vi "Initialize.vi"(8 "error in (no error)":errorcluster, 9 "Reset? ( Yes)":bool=TRUE, 10 "ID Query? ( Yes)":bool=TRUE, 11 "VISA resource name":refnum<visa-resource-name>) -> (0 "error out":errorcluster, 3 "VISA resource name out":refnum<visa-resource-name>)   [LabVIEW 2011, in "Tektronix 7000 Series.lvlib"]
doc: "Establishes communication with the instrument and optionally performs an instrument identification query or an instrument reset. This VI also places the instrument in a default state needed for other instrument driver operations.\nRun this VI before running other instrument driver VIs for the instrument. You generally need to run the Initialize VI only once, at the beginning of an application."
uses:
  Tektronix 7000 Series.lvlib
panel:
  # "Copyright 2006 - 2011 National Instruments Corporation.  ALL RIGHTS RESERVED."
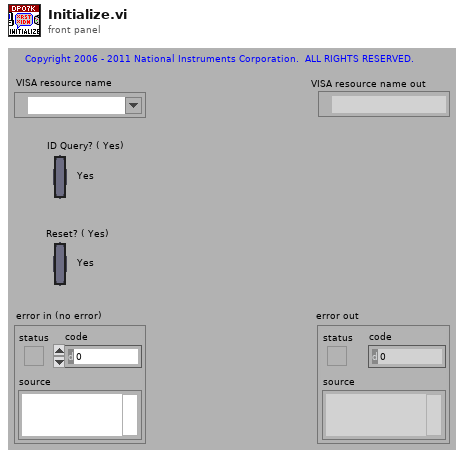
[diagram p1: front panel]
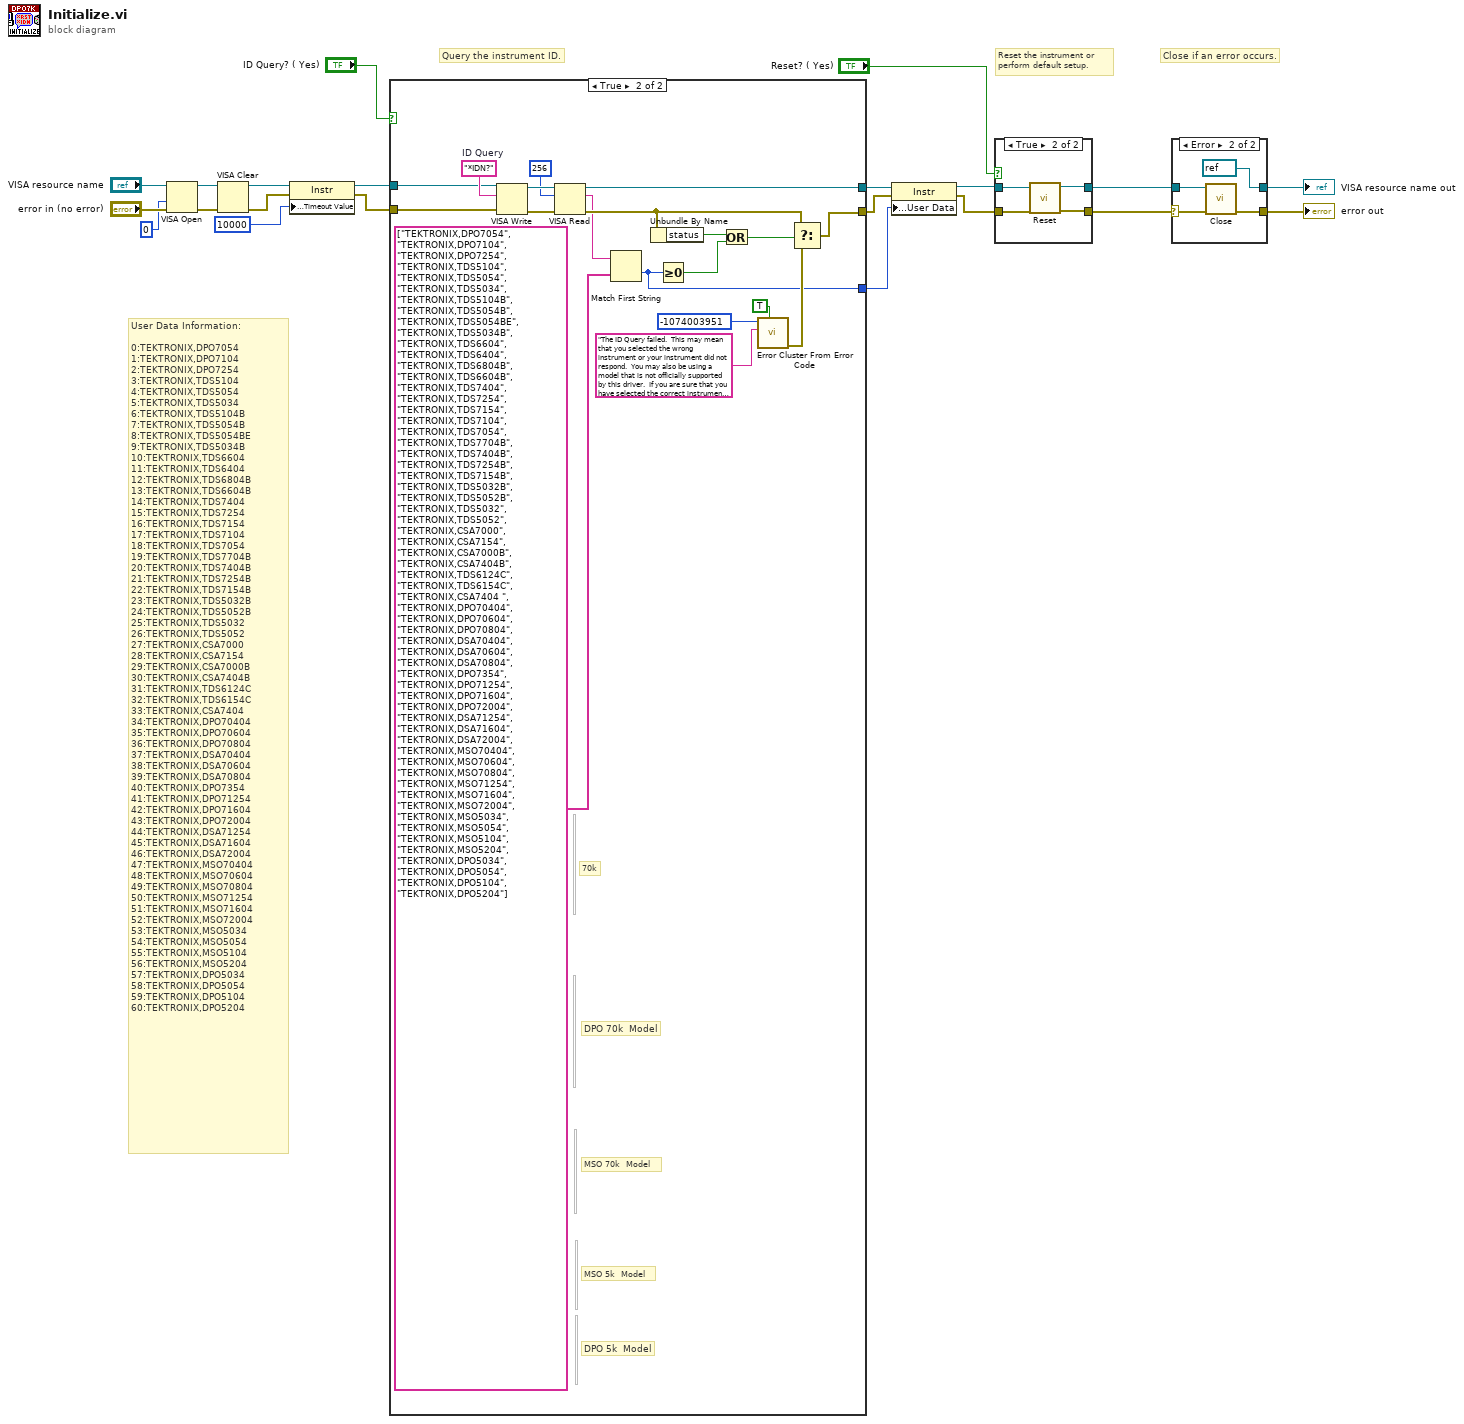
[diagram p0: block diagram]
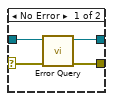
[diagram p2: hidden frame]
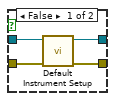
[diagram p3: hidden frame]
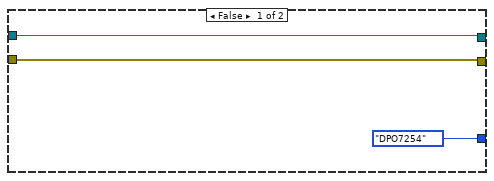
[diagram p4: hidden frame]
diagram:
  # "User Data Information:\n\n0:TEKTRONIX,DPO7054\n1:TEKTRONIX,DPO7104\n2:TEKTRONIX,DPO7254\n3:TEKTRONIX,TDS5104\n4:TEKTRONIX,TDS5054\n5:TEKTRONIX,TDS5034\n6:TEKTRONIX,TDS5104B\n7:TEKTRONIX,TDS5054B\n8:TEKTRONIX,TDS5054BE\n9:TEKTRONIX,TDS5034B\n10:TEKTRONIX,TDS6604\n11:TEKTRONIX,TDS6404\n12:TEKTRONIX,TDS6804B\n13:TEKTRONIX,TDS6604B\n14:TEKTRONIX,TDS7404\n15:TEKTRONIX,TDS7254\n16:TEKTRONIX,TDS7154\n17:TEKTRONIX,TDS7104\n18:TEKTRONIX,TDS7054\n19:TEKTRONIX,TDS7704B\n20:TEKTRONIX,TDS7404B\n21:TEKTRONIX,TDS7254B\n22:TEKTRONIX,TDS7154B\n23:TEKTRONIX,TDS5032B\n24:TEKTRONIX,TDS5052B\n25:TEKTRONIX,TDS5032\n26:TEKTRONIX,TDS5052\n27:TEKTRONIX,CSA7000\n28:TEKTRONIX,CSA7154\n29:TEKTRONIX,CSA7000B\n30:TEKTRONIX,CSA7404B\n31:TEKTRONIX,TDS6124C\n32:TEKTRONIX,TDS6154C\n33:TEKTRONIX,CSA7404\n34:TEKTRONIX,DPO70404\n35:TEKTRONIX,DPO70604\n36:TEKTRONIX,DPO70804\n37:TEKTRONIX,DSA70404\n38:TEKTRONIX,DSA70604\n39:TEKTRONIX,DSA70804\n40:TEKTRONIX,DPO7354\n41:TEKTRONIX,DPO71254\n42:TEKTRONIX,DPO71604\n43:TEKTRONIX,DPO72004\n44:TEKTRONIX,DSA71254\n45:TEKTRONIX,DSA71604\n46:TEKTRONIX,DSA72004\n47:TEKTRONIX,MSO70404\n48:TEKTRONIX,MSO70604\n49:TEKTRONIX,MSO70804\n50:TEKTRONIX,MSO71254\n51:TEKTRONIX,MSO71604\n52:TEKTRONIX,MSO72004\n53:TEKTRONIX,MSO5034\n54:TEKTRONIX,MSO5054\n55:TEKTRONIX,MSO5104\n56:TEKTRONIX,MSO5204\n57:TEKTRONIX,DPO5034\n58:TEKTRONIX,DPO5054\n59:TEKTRONIX,DPO5104\n60:TEKTRONIX,DPO5204"
  # "Close if an error occurs."
  # "Query the instrument ID."
  # "Reset the instrument or\nperform default setup."
  n1 = VISA Open(access mode=u32 0, error in (no error)="error in (no error)", VISA resource name="VISA resource name") -> (VISA resource name=w16:refnum<visa-resource-name>, error out=w15:errorcluster)  [unwired: 2 in]
  n2 = VISA Clear(VISA resource name=w16, error in (no error)=w15) -> (VISA resource name out=w3:refnum<visa-resource-name>, error out=w2:errorcluster)
  n3 = property on="Property Node" class="Instr"(reference=w3, error in=w2, "General Settings:Timeout Value"=u32 10000) -> (reference out=w5:refnum<visa-resource-name>, error out=w4:errorcluster)
  n4 = case shown="True" "ID Query? ( Yes)" {
    tunnel: [w23 w43] -> w10
    tunnel: [w24 w42] -> w6
    tunnel: w5 -> [w24 w29]
    tunnel: w4 -> [w23 w28]
    tunnel: [enum16{"DPO7054", "DPO7104", "DPO7254"}."DPO7254" w26] -> w7
    frame False {
    }
    frame True {
      w38 = "*IDN?"  # ID Query
      # "60"
      # "59"
      # "58"
      # "57"
      # "DPO 5k  Model"
      # "MSO 5k  Model"
      # "56"
      # "55"
      # "54"
      # "53"
      # "MSO 70k  Model"
      # "52"
      # "51"
      # "50"
      # "49"
      # "48"
      # "47"
      # "46"
      # "45"
      # "44"
      # "43"
      # "42"
      # "41"
      # "40"
      # "DPO 70k  Model"
      # "70k"
      # "39"
      # "38"
      # "37"
      # "36"
      # "35"
      # "34"
      # "33"
      # "32"
      # "31"
      # "30"
      # "29"
      # "28"
      # "27"
      # "26"
      # "25"
      # "24"
      # "23"
      # "22"
      # "21"
      # "20"
      # "19"
      # "18"
      # "17"
      # "16"
      # "15"
      # "14"
      # "13"
      # "12"
      # "11"
      # "10"
      # "9"
      # "8"
      # "7"
      # "6"
      # "5"
      # "4"
      # "3"
      # "2"
      # "1"
      n5 = VISA Write(VISA resource name=w29, write buffer=w38, error in (no error)=w28) -> (VISA resource name out=w41:refnum<visa-resource-name>, error out=w40:errorcluster)  [unwired: 1 out]
      n6 = VISA Read(VISA resource name=w41, byte count=u32 256, error in (no error)=w40) -> (VISA resource name out=w42:refnum<visa-resource-name>, read buffer=w27:string, error out=w33:errorcluster)  [unwired: 1 out]
      n7 = Match First String(2:string[] ["TEKTRONIX,DPO7054", "TEKTRONIX,DPO7104", "TEKTRONIX,DPO7254", "TEKTRONIX,TDS5104", "TEKTRONIX,TDS5054", "TEKTRONIX,TDS5034", "TEKTRONIX,TDS5104B", "TEKTRONIX,TDS5054B", "TEKTRONIX,TDS5054BE", "TEKTRONIX,TDS5034B", "TEKTRONIX,TDS6604", "TEKTRONIX,TDS6404", "TEKTRONIX,TDS6804B", "TEKTRONIX,TDS6604B", "TEKTRONIX,TDS7404", "TEKTRONIX,TDS7254", "TEKTRONIX,TDS7154", "TEKTRONIX,TDS7104", "TEKTRONIX,TDS7054", "TEKTRONIX,TDS7704B", "TEKTRONIX,TDS7404B", "TEKTRONIX,TDS7254B", "TEKTRONIX,TDS7154B", "TEKTRONIX,TDS5032B", "TEKTRONIX,TDS5052B", "TEKTRONIX,TDS5032", "TEKTRONIX,TDS5052", "TEKTRONIX,CSA7000", "TEKTRONIX,CSA7154", "TEKTRONIX,CSA7000B", "TEKTRONIX,CSA7404B", "TEKTRONIX,TDS6124C", "TEKTRONIX,TDS6154C", "TEKTRONIX,CSA7404 ", "TEKTRONIX,DPO70404", "TEKTRONIX,DPO70604", "TEKTRONIX,DPO70804", "TEKTRONIX,DSA70404", "TEKTRONIX,DSA70604", "TEKTRONIX,DSA70804", "TEKTRONIX,DPO7354", "TEKTRONIX,DPO71254", "TEKTRONIX,DPO71604", "TEKTRONIX,DPO72004", "TEKTRONIX,DSA71254", "TEKTRONIX,DSA71604", "TEKTRONIX,DSA72004", "TEKTRONIX,MSO70404", "TEKTRONIX,MSO70604", "TEKTRONIX,MSO70804", "TEKTRONIX,MSO71254", "TEKTRONIX,MSO71604", "TEKTRONIX,MSO72004", "TEKTRONIX,MSO5034", "TEKTRONIX,MSO5054", "TEKTRONIX,MSO5104", "TEKTRONIX,MSO5204", "TEKTRONIX,DPO5034", "TEKTRONIX,DPO5054", "TEKTRONIX,DPO5104", "TEKTRONIX,DPO5204"], 3:w27) -> (0:w26:i32)  [unwired: 1 out]
      n8 = Unbundle By Name(w33) -> ("status"=w31:bool)
      n9 = Greater Or Equal To 0?(x=w26) -> (x >= 0?=w30:bool)
      n10 = Or(x=w31, y=w30) -> (x .or. y?=w32:bool)
      n11 = call <vilib>:"Error Cluster From Error Code.vi"("show call chain? (False)"=TRUE, "error message (\"\")"="The ID Query failed.  This may mean that you selected the wrong instrument or your instrument did not respond.  You may also be using a model that is not officially supported by this driver.  If you are sure that you have selected the correct instrument and it is responding, try disabling the ID Query." ("Source (VI Name)"), "error code (0)"=-1074003951 ("Code")) -> ("error out"=w37:errorcluster)  [unwired: 6 in]
      n12 = Select(t=w33, s=w32, f=w37) -> (s? t:f=w43:errorcluster)
    }
  }
  n13 = property class="Instr"(reference=w6, error in=w10, "General Settings:User Data"=w7) -> (reference out=w9:refnum<visa-resource-name>, error out=w8:errorcluster)
  n14 = case shown="True" "Reset? ( Yes)" {
    tunnel: w8 -> [w45 w50]
    tunnel: [w44 w48] -> w11
    tunnel: w9 -> [w47 w51]
    tunnel: [w46 w49] -> w12
    frame False {
      n15 = call "Default Instrument Setup.vi"("error in (no error)"=w45, "VISA resource name"=w47) -> ("error out"=w44:errorcluster, "VISA resource name out"=w46:refnum<visa-resource-name>)  [unwired: 8 in]
    }
    frame True {
      n16 = call "Reset.vi"("error in (no error)"=w50, "VISA resource name"=w51) -> ("error out"=w48:errorcluster, "VISA resource name out"=w49:refnum<visa-resource-name>)  [unwired: 8 in]
    }
  }
  n17 = case shown="Error" w11 {
    selector: w11 -> [w53 w57]
    tunnel: w12 -> [w52 w58]
    tunnel: [w55 refnum<visa-resource-name> refnum ("VISA resource name out")] -> w14
    tunnel: [w54 w59] -> w13
    frame No Error {
      n18 = call "Error Query.vi"("error in (no error)"=w53, "VISA resource name"=w52) -> ("error out"=w54:errorcluster, "VISA resource name out"=w55:refnum<visa-resource-name>)  [unwired: 6 in, 2 out]
    }
    frame Error {
      n19 = call "Close.vi"("error in (no error)"=w57, "VISA resource name"=w58) -> ("error out"=w59:errorcluster)  [unwired: 9 in]
    }
  }
  "VISA resource name out" <- w14
  "error out" <- w13
